vi "Interpret_LiDAR_Ray_Header.vi"(11 "Data in":u8[](array[numeric])) -> (2 "Ray Data out":T1 {"Return Data Array"."Reflectance" format="%.6f %"; "Return Data Array"."Range" format="%.4f M"; "Return Data Array"."Existence Probability" format="%.4f %"; "Elevation" format="%.6f"; "Azimuth" format="%.6f"}, 3 "Remaining Data out":u8[](array[numeric]))   [LabVIEW 2018, in "LiDAR.lvlib" / "LiDAR.lvclass"]
uses:
  LiDAR.lvclass
  Controls/cls_Point_Cloud_Ray_Header.ctl
  Controls/cls_Point_Cloud_Return_Data.ctl
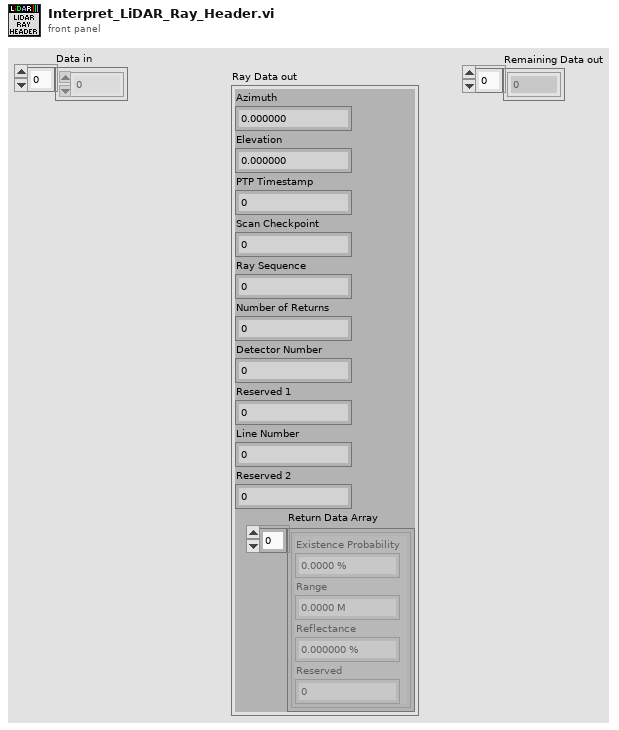
[diagram p1: front panel]
types:
  T1 = typedef "LiDAR.lvlib/LiDAR.lvclass/cls_Point_Cloud_Ray_Header.ctl" = cluster{"Azimuth":dbl, "Elevation":dbl, "PTP Timestamp":u32, "Scan Checkpoint":u8, "Ray Sequence":u8, "Number of Returns":u8, "Detector Number":u8, "Reserved 1":u8, "Line Number":u16, "Reserved 2":u32, "Return Data Array":T2[]}
  T2 = typedef "LiDAR.lvlib/LiDAR.lvclass/cls_Point_Cloud_Return_Data.ctl" = cluster{"Existence Probability":dbl, "Range":dbl, "Reflectance":dbl, "Reserved":u16}
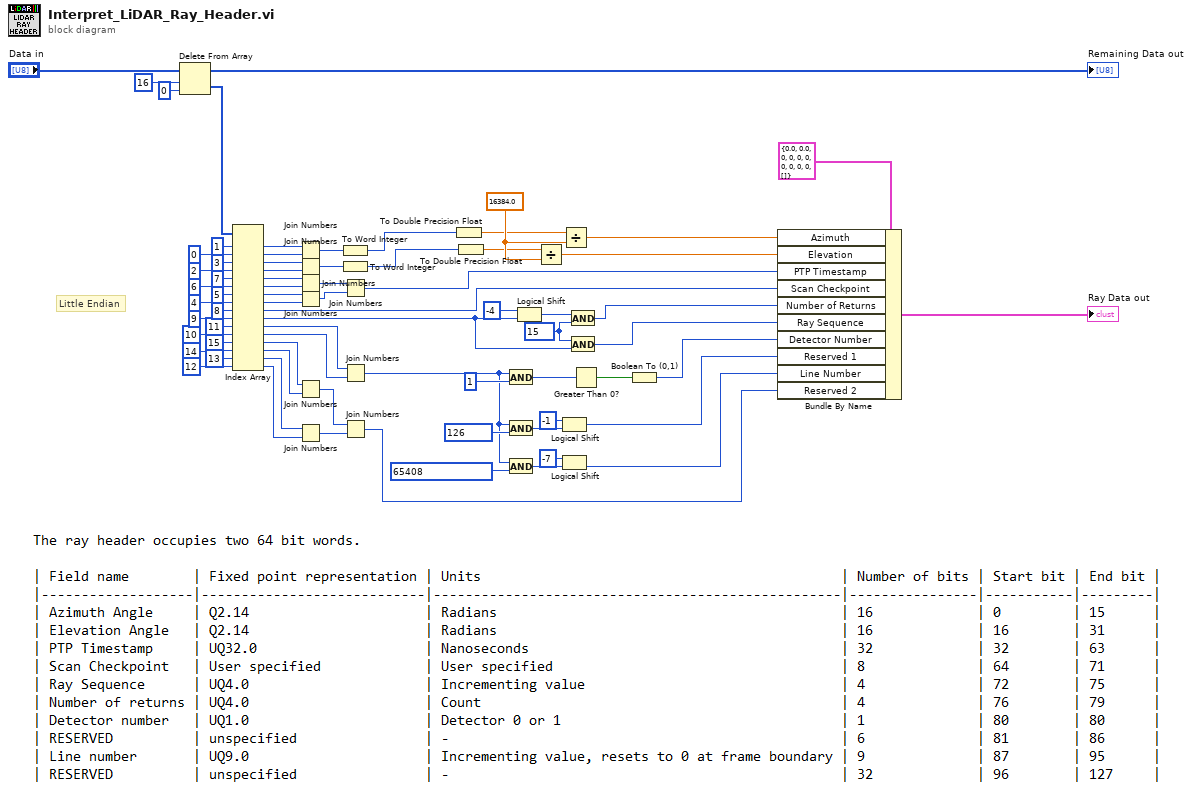
[diagram p0: block diagram]
diagram:
  w5 = 16384.0
  w36 = u8 15 ("y")
  # "Little Endian"
  n1 = Delete From Array(array="Data in", length=16, index=0) -> (deleted portion=w69:u8[], array with subset deleted=→"Remaining Data out":u8[])
  n2 = Index Array(array=w69, index #1=1 ("index"), index #2=0 ("index"), index #3=3 ("index"), index #4=2 ("index"), index #5=7 ("index"), index #6=6 ("index"), index #7=5 ("index"), index #8=4 ("index"), index #9=8 ("index"), index #10=9 ("index"), index #11=11 ("index"), index #12=10 ("index"), index #13=15 ("index"), index #14=14 ("index"), index #15=13 ("index"), index #16=12 ("index")) -> (element #1=w33:u8, element #2=w30:u8, element #3=w32:u8, element #4=w31:u8, element #5=w68:u8, element #6=w67:u8, element #7=w66:u8, element #8=w65:u8, element #9=w61:u8, element #10=w39:u8, element #11=w60:u8, element #12=w59:u8, element #13=w49:u8, element #14=w48:u8, element #15=w47:u8, element #16=w46:u8)
  n3 = Join Numbers(hi=w33, lo=w30) -> ((hi.lo)=w8:u16)
  n4 = Join Numbers(hi=w32, lo=w31) -> ((hi.lo)=w9:u16)
  n5 = Join Numbers(hi=w68, lo=w67) -> ((hi.lo)=w63:u16)
  n6 = Join Numbers(hi=w66, lo=w65) -> ((hi.lo)=w64:u16)
  n7 = Join Numbers(hi=w49, lo=w48) -> ((hi.lo)=w44:u16)
  n8 = Join Numbers(hi=w47, lo=w46) -> ((hi.lo)=w45:u16)
  n9 = To Word Integer(number=w8) -> (16bit integer=w7:i16)
  n10 = To Word Integer(number=w9) -> (16bit integer=w6:i16)
  n11 = Join Numbers(hi=w63, lo=w64) -> ((hi.lo)=w62:u32)
  n12 = Join Numbers(hi=w60, lo=w59) -> ((hi.lo)=w52:u16)
  n13 = Join Numbers(hi=w44, lo=w45) -> ((hi.lo)=w43:u32)
  n14 = To Double Precision Float(number=w7) -> (double precision float=w1:dbl)
  n15 = To Double Precision Float(number=w6) -> (double precision float=w2:dbl)
  n16 = And(x=w52, y=u16 1) -> (x .and. y?=w56:u16)
  n17 = And(x=w52, y=u16 126) -> (x .and. y?=w12:u16)
  n18 = And(x=w52, y=u16 65408) -> (x .and. y?=w50:u16)
  n19 = Logical Shift(y=i16 -4, x=w39) -> (x << y=w37:u8)
  n20 = Divide(x=w2, y=w5) -> (x/y=w3:dbl)
  n21 = Logical Shift(y=i16 -1, x=w12) -> (x << y=w10:u16)
  n22 = Logical Shift(y=i16 -7, x=w50) -> (x << y=w14:u16)
  n23 = Divide(x=w1, y=w5) -> (x/y=w4:dbl)
  n24 = And(x=w37, y=w36) -> (x .and. y?=w35:u8)
  n25 = And(x=w36, y=w39) -> (x .and. y?=w34:u8)
  n26 = Greater Than 0?(x=w56) -> (x > 0?=w55:bool)
  n27 = Boolean To (0,1)(Boolean=w55) -> (0, 1=w54:i16)
  n28 = Bundle By Name(cluster=T1 {"Azimuth"=0.0, "Elevation"=0.0, "PTP Timestamp"=0, "Scan Checkpoint"=0, "Ray Sequence"=0, "Number of Returns"=0, "Detector Number"=0, "Reserved 1"=0, "Line Number"=0, "Reserved 2"=0, "Return Data Array"=[]} ("Point Cloud Ray Header"), "Azimuth"=w4, "Elevation"=w3, "PTP Timestamp"=w62, "Scan Checkpoint"=w61, "Number of Returns"=w35, "Ray Sequence"=w34, "Detector Number"=w54, "Reserved 1"=w10, "Line Number"=w14, "Reserved 2"=w43) -> (→"Ray Data out":T1)
